vi "PPL RT Driver VI_InlineHW.vi"(7 "Operation":T1, 11 "Device Reference in":T2 format="%.0x") -> (0 "Error Code":i32)   [LabVIEW 2020]
uses:
  <vilib>/NI VeriStand/Custom Device API/Custom Device Item Ref.ctl
  <vilib>/NI VeriStand/Custom Device API/Hardware Interface Driver VI Operation.ctl
  <vilib>/NI VeriStand/Custom Device API/Custom Device Channel Type.ctl
  <vilib>/NI VeriStand/Custom Device API/Data Reference.ctl
  <vilib>/NI VeriStand/Custom Device API/Data Access Type.ctl
  <vilib>/NI VeriStand/Custom Device API/Global Data Refs.vi
  <vilib>/NI VeriStand/Custom Device API/Custom Device API.lvlib
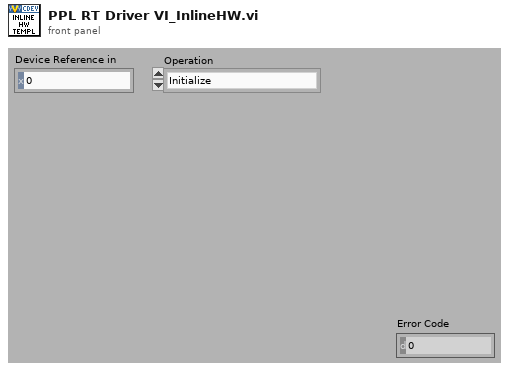
[diagram p1: front panel]
types:
  T1 = typedef "Custom Device API.lvlib/Hardware Interface Driver VI Operation.ctl" = enum16{"Initialize", "Start", "Read Data from HW", "Write Data to HW", "Close"}
  T2 = typedef "Custom Device API.lvlib/Custom Device Item Ref.ctl" = u64
  T3 = typedef "Custom Device API.lvlib/Data Reference.ctl" = i32
  T4 = cluster{"Input Values":dbl[], "Input Refs":T3[], "Output Values":dbl[], "Output Refs":T3[], "Device Error":errorcluster}
  T5 = typedef "Custom Device API.lvlib/Custom Device Channel Type.ctl" = enum16{"Input", "Output"}
  T6 = typedef "Custom Device API.lvlib/Data Access Type.ctl" = enum16{"Read", "Write"}
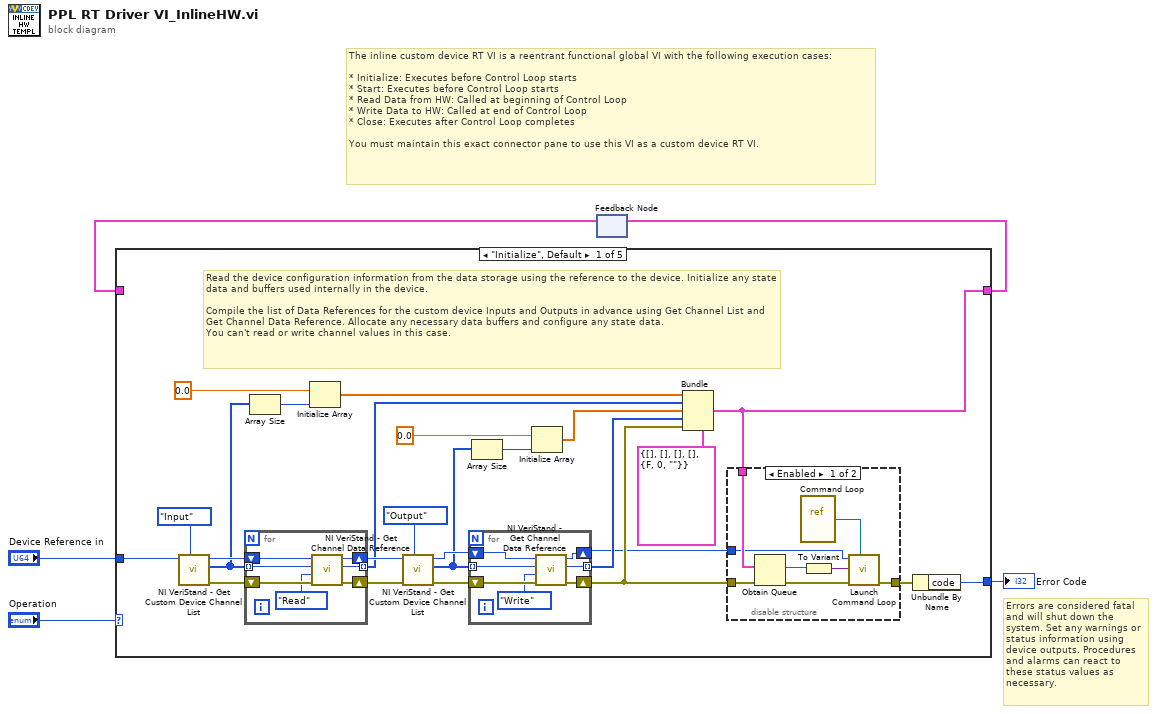
[diagram p0: block diagram]
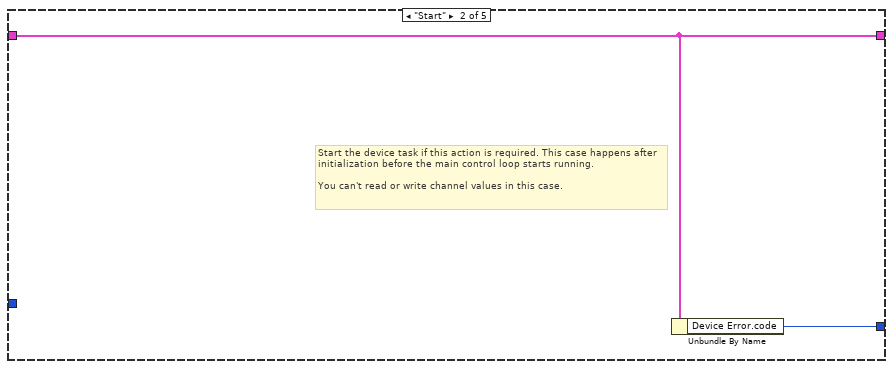
[diagram p3: hidden frame]
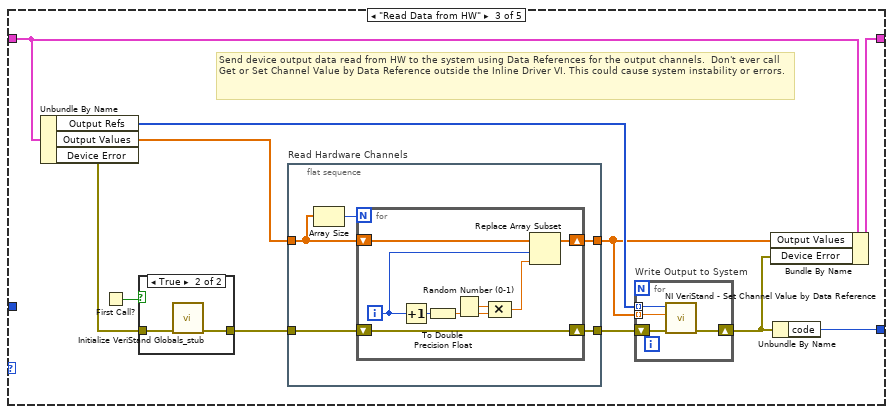
[diagram p4: hidden frame]
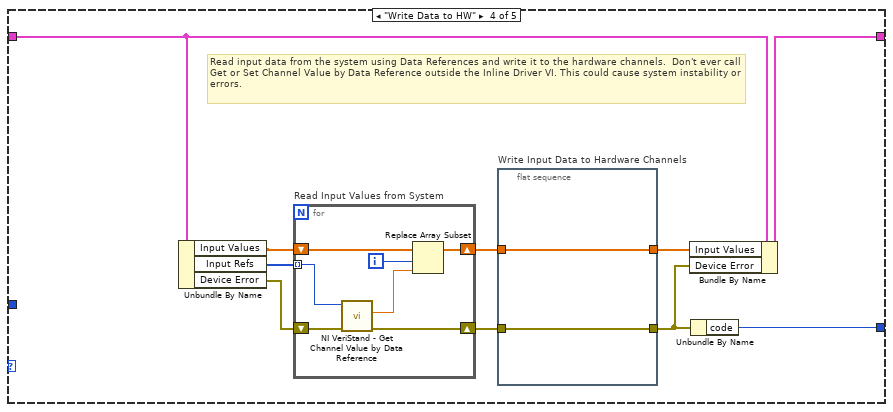
[diagram p6: hidden frame]
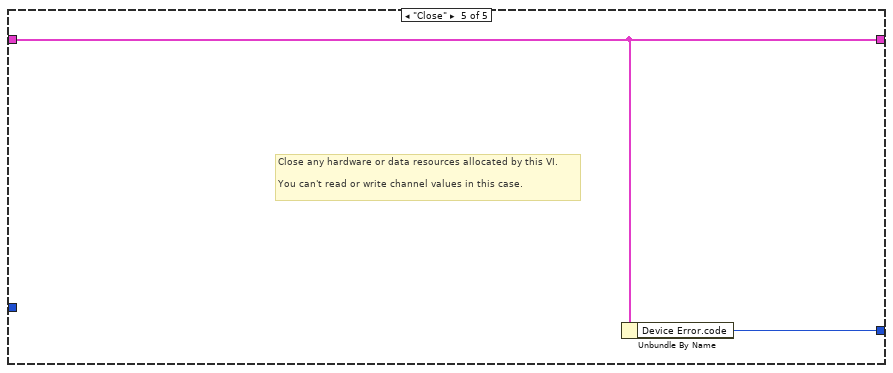
[diagram p7: hidden frame]
diagram:
  # "Errors are considered fatal and will shut down the system. Set any warnings or status information using device outputs. Procedures and alarms can react to these status values as necessary."
  # "The inline custom device RT VI is a reentrant functional global VI with the following execution cases:\n\n* Initialize: Executes before Control Loop starts\n* Start: Executes before Control Loop starts\n* Read Data from HW: Called at beginning of Control Loop\n* Write Data to HW: Called at end of Control Loop\n* Close: Executes after Control Loop completes\n\nYou must maintain this exact connector pane to use this VI as a custom device RT VI."
  n1 = feedback #1() -> (w3:T4)  [unwired: 1 out]
  n2 = case shown="\"Initialize\", Default" "Operation" {
    tunnel: [w9 w54 w61 w95 w106] -> w4
    tunnel: w3 -> [_ w54 w62 w96 w106]
    tunnel: "Device Reference in" -> [w26 _ _ _ _]
    tunnel: [w25 w55 w65 w89 w107] -> w1
    frame "Initialize", Default {
      # "Read the device configuration information from the data storage using the reference to the device. Initialize any state data and buffers used internally in the device.\n\nCompile the list of Data References for the custom device Inputs and Outputs in advance using Get Channel List and Get Channel Data Reference. Allocate any necessary data buffers and configure any state data.\nYou can't read or write channel values in this case."
      n3 = call <vilib>:"NI VeriStand - Get Custom Device Channel List.vi"("Channel Type"=Custom_Device_Channel_Type."Input", "Device Ref in"=w26) -> ("error out"=w23:errorcluster, "Specified Channel Ref List"=w22:T2[], "Device Ref out"=w24:T2)  [unwired: 1 in, 6 out]
      n4 = for {
        shift-right: [w48] -> w18
        shift-left: w24 -> [w52]
        tunnel: w22 -> [w51] mode=indexing
        shift-right: [w49] -> w17
        shift-left: w23 -> [w53]
        tunnel: [w47] -> w16 mode=indexing
        n5 = call <vilib>:"NI VeriStand - Get Channel Data Reference.vi"("error in (no error)"=w53, "Access"=Data_Access_Type."Read", "Channel Ref in"=w51, "Device Ref in"=w52) -> ("error out"=w49:errorcluster, "Channel Data Reference"=w47:T3, "Device Ref out"=w48:T2)  [unwired: 5 out]
      }
      n6 = Array Size(array=w22) -> (size(s)=w29:i32)
      n7 = Initialize Array(0.0 ("element"), w29) -> (w30:dbl[])
      n8 = call <vilib>:"NI VeriStand - Get Custom Device Channel List.vi"("Channel Type"=Custom_Device_Channel_Type."Output", "error in (no error)"=w17, "Device Ref in"=w18) -> ("error out"=w21:errorcluster, "Specified Channel Ref List"=w13:T2[], "Device Ref out"=w20:T2)  [unwired: 6 out]
      n9 = for {
        tunnel: w13 -> [w44] mode=indexing
        shift-right: [w42] -> w8
        shift-left: w21 -> [w46]
        tunnel: [w41] -> w11 mode=indexing
        shift-right: [w40] -> w6
        shift-left: w20 -> [w45]
        n10 = call <vilib>:"NI VeriStand - Get Channel Data Reference.vi"("error in (no error)"=w46, "Access"=Data_Access_Type."Write", "Channel Ref in"=w44, "Device Ref in"=w45) -> ("error out"=w42:errorcluster, "Channel Data Reference"=w41:T3, "Device Ref out"=w40:T2)  [unwired: 5 out]
      }
      n11 = Array Size(array=w13) -> (size(s)=w14:i32)
      n12 = Initialize Array(0.0 ("element"), w14) -> (w12:dbl[])
      n13 = Bundle(cluster=T4 {"Input Values"=[], "Input Refs"=[], "Output Values"=[], "Output Refs"=[], "Device Error"={"status"=FALSE, "code"=0, "source"=""}}, "Input Values"=w30, "Input Refs"=w16, "Output Values"=w12, "Output Refs"=w11, "Device Error"=w8) -> (w9:T4)
      n14 = disable-structure shown="Enabled" {
        disable-tunnel: w9 -> [w38 _]
        disable-tunnel: w8 -> [w35 w39]
        disable-tunnel: [w33 w39] -> w7
        disable-tunnel: w6 -> [w31 _]
        frame Enabled {
          n15 = Obtain Queue(element data type=w38, error in (no error)=w35) -> (queue out=w37:refnum<queue>, error out=w34:errorcluster)  [unwired: 3 in, 1 out]
          n16 = vi-ref "Command Loop.vi"() -> (w32:refnum<vi>)
          n17 = To Variant(anything=w37) -> (Variant=w36:variant)
          n18 = call "Launch Command Loop.vi"("VI Refnum"=w32, "error in"=w34, "Queue Refs"=w36, "Device Reference in"=w31) -> ("error out"=w33:errorcluster)  [unwired: 7 in]
        }
        frame Disabled {
        }
      }
      n19 = Unbundle By Name(w7) -> ("code"=w25:i32)
    }
    frame "Start" {
      # "Start the device task if this action is required. This case happens after initialization before the main control loop starts running.\n\nYou can't read or write channel values in this case."
      n20 = Unbundle By Name(w54) -> ("Device Error.code"=w55:i32)
    }
    frame "Read Data from HW" {
      # "Send device output data read from HW to the system using Data References for the output channels.  Don't ever call Get or Set Channel Value by Data Reference outside the Inline Driver VI. This could cause system instability or errors."
      n21 = Unbundle By Name(w62) -> ("Output Refs"=w64:T3[], "Output Values"=w63:dbl[], "Device Error"=w56:errorcluster)
      n22 = First Call?() -> (First Call?: T/F=w58:bool)
      n23 = case shown="True" w58 {
        tunnel: [w67 w68] -> w57
        tunnel: w56 -> [w67 w69]
        frame False {
        }
        frame True {
          n24 = call "Initialize VeriStand Globals_stub.vi"("error in (no error)"=w69) -> ("error out"=w68:errorcluster)  [unwired: 10 in]
        }
      }
      n25 = flat-sequence "Read Hardware Channels" {
        tunnel: w57 -> [w78]
        tunnel: [w77] -> w66
        tunnel: [w74] -> w60
        tunnel: w63 -> [w75]
        frame #0 {
          n26 = Array Size(array=w75) -> (size(s)=w76:i32)
          n27 = for {
            N: w76 -> [_]
            shift-right: [w83] -> w77
            shift-left: w78 -> [w83]
            shift-right: [w80] -> w74
            shift-left: w75 -> [w82]
            i -> [w79]
            n28 = Increment(x=w79) -> (x+1=w85:i32)
            n29 = To Double Precision Float(number=w85) -> (double precision float=w84:dbl)
            n30 = Random Number (0-1)() -> (number: 0 to 1=w86:dbl)
            n31 = Compound Arithmetic op=MULTIPLY(w86, w84) -> (w81:dbl)
            n32 = Replace Array Subset(array=w82, new element=w81, index=w79) -> (w80:dbl[])
          }
        }
      }
      n33 = for "Write Output to System" {
        shift-right: [w72] -> w59
        shift-left: w66 -> [w73]
        tunnel: w60 -> [w71] mode=indexing
        tunnel: w64 -> [w70] mode=indexing
        n34 = call <vilib>:"NI VeriStand - Set Channel Value by Data Reference.vi"("error in (no error)"=w73, "Value"=w71, "Data Reference in"=w70) -> ("error out"=w72:errorcluster)  [unwired: 8 out]
      }
      n35 = Bundle By Name(cluster=w62, "Output Values"=w60, "Device Error"=w59) -> (w61:T4)
      n36 = Unbundle By Name(w59) -> ("code"=w65:i32)
    }
    frame "Write Data to HW" {
      # "Read input data from the system using Data References and write it to the hardware channels.  Don't ever call Get or Set Channel Value by Data Reference outside the Inline Driver VI. This could cause system instability or errors."
      n37 = Unbundle By Name(w96) -> ("Input Values"=w93:dbl[], "Input Refs"=w94:T3[], "Device Error"=w88:errorcluster)
      n38 = for "Read Input Values from System" {
        shift-right: [w99] -> w90
        shift-left: w88 -> [w105]
        tunnel: w94 -> [w104] mode=indexing
        shift-right: [w102] -> w92
        shift-left: w93 -> [w103]
        i -> [w101]
        n39 = call <vilib>:"NI VeriStand - Get Channel Value by Data Reference.vi"("error in (no error)"=w105, "Data Reference in"=w104) -> ("error out"=w99:errorcluster, "Value"=w100:dbl)  [unwired: 8 out]
        n40 = Replace Array Subset(array=w103, new element=w100, index=w101) -> (w102:dbl[])
      }
      n41 = flat-sequence "Write Input Data to Hardware Channels" {
        tunnel: w92 -> [w98]
        tunnel: [w98] -> w91
        tunnel: [w97] -> w87
        tunnel: w90 -> [w97]
        frame #0 {
        }
      }
      n42 = Bundle By Name(cluster=w96, "Input Values"=w91, "Device Error"=w87) -> (w95:T4)
      n43 = Unbundle By Name(w87) -> ("code"=w89:i32)
    }
    frame "Close" {
      # "Close any hardware or data resources allocated by this VI.\n\nYou can't read or write channel values in this case."
      n44 = Unbundle By Name(w106) -> ("Device Error.code"=w107:i32)
    }
  }
  "Error Code" <- w1
  n45 = feedback-in #1(w4) -> ()
